vi "Emphasize Colo2r.vi"(2 "error in (no error)":errorcluster, 3 "Color":i8, 4 "Image Dst":T1, 5 "Image Src":T1) -> (0 "error out":errorcluster, 1 "Image Out":T1)   [LabVIEW 2009, in "ImageProcessing.lvlib"]
doc: "Output is a grayscaled image calculated as\n (255*X)/(R+G+B) \nwhere X is R, G or B depending on what number is showsen in color (0 = R, 1 = G, 2 = B)."
uses:
  ImageProcessing.lvlib
  <vilib>/vision/Image Controls.llb/IMAQ Image.ctl
  <vilib>/Analysis/Matrix/Numeric/Conversions/Matrix To Array - RM.vi
  <vilib>/Analysis/Matrix/Numeric/Multiply/Multiply - RM,R.vi
  <vilib>/Analysis/Matrix/Numeric/Add/Add - RM,RM.vi
  <vilib>/Analysis/Matrix/Numeric/Conversions/Array To Matrix - RA2.vi
  <vilib>/Analysis/Matrix/NI_Matrix.lvlib
  <vilib>/vision/NI_Vision_Development_Module.lvlib
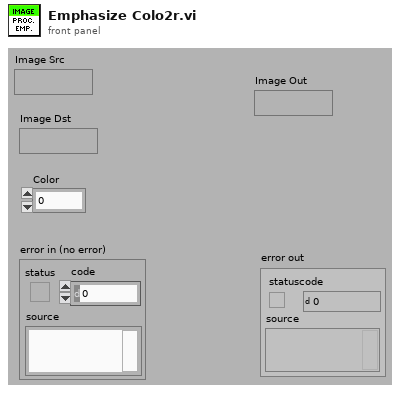
[diagram p1: front panel]
types:
  T1 = typedef "IMAQ Image.ctl" = refnum<image>
  T2 = typedef "NI_Matrix.lvlib/RealMatrix.ctl" = dbl[][]
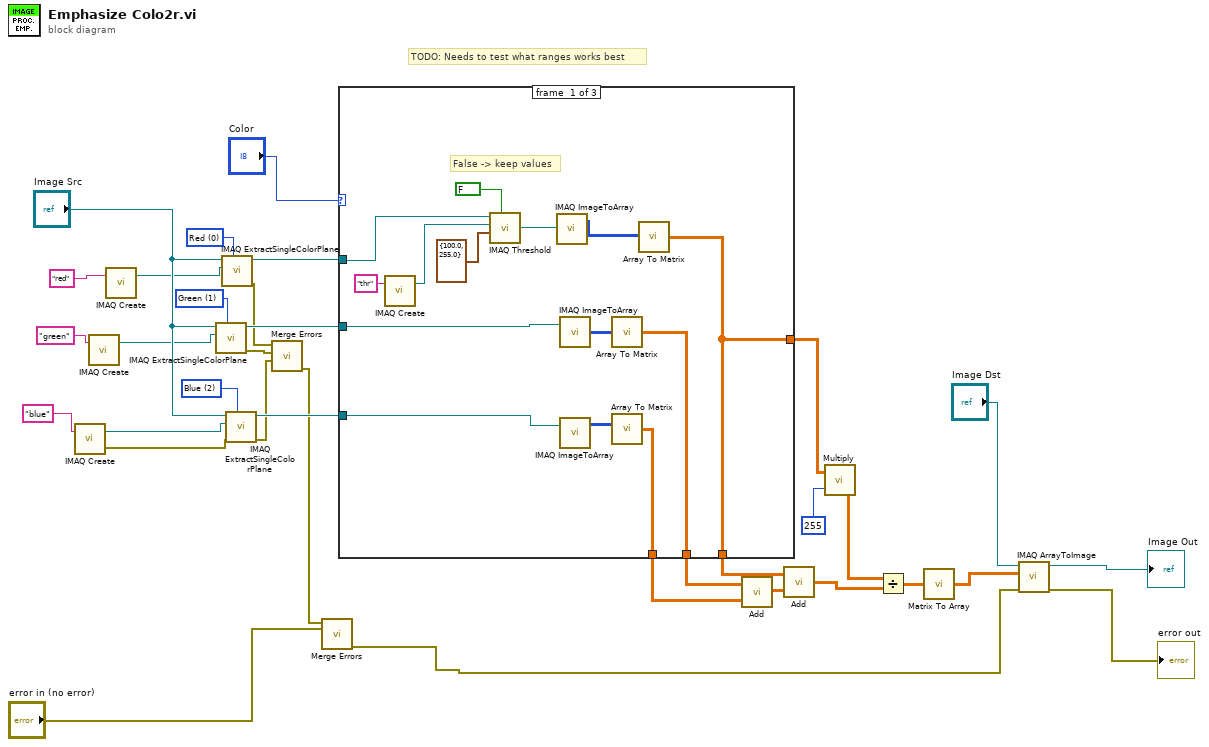
[diagram p0: block diagram]
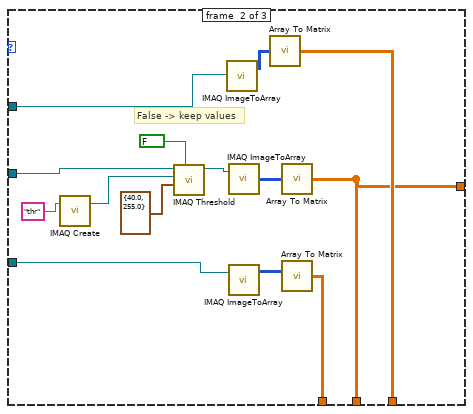
[diagram p2: hidden frame]
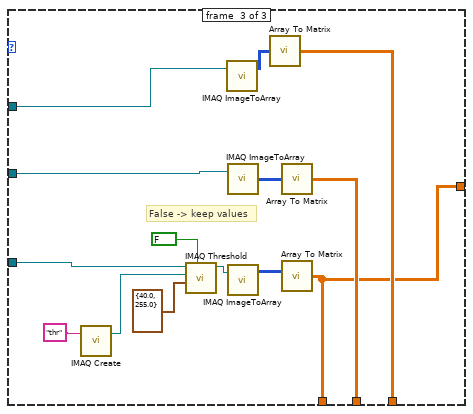
[diagram p3: hidden frame]
diagram:
  w22 = 2 items=["Red", "Green", "Blue", "Hue", "Saturation", "Luminance", "Value", "Intensity"] ("Color Plane")
  w21 = 1 items=["Red", "Green", "Blue", "Hue", "Saturation", "Luminance", "Value", "Intensity"] ("Color Plane")
  w20 = 0 items=["Red", "Green", "Blue", "Hue", "Saturation", "Luminance", "Value", "Intensity"] ("Color Plane")
  # "TODO: Needs to test what ranges works best"
  n1 = call "IMAQ Create"("Image Name"="blue") -> ("New Image"=w16:T1, "error out"=w10:errorcluster)  [unwired: 3 in, 1 out]
  n2 = call "IMAQ Create"("Image Name"="green") -> ("New Image"=w17:T1)  [unwired: 3 in, 2 out]
  n3 = call "IMAQ Create"("Image Name"="red") -> ("New Image"=w18:T1)  [unwired: 3 in, 2 out]
  n4 = call "IMAQ ExtractSingleColorPlane"("Color Plane"=w21, "Image Dst"=w17, "Image Src"="Image Src") -> ("error out"=w8:errorcluster, "Image Dst Out"=w15:T1)  [unwired: 7 in]
  n5 = call "IMAQ ExtractSingleColorPlane"("Color Plane"=w20, "Image Dst"=w18, "Image Src"="Image Src") -> ("error out"=w7:errorcluster, "Image Dst Out"=w3:T1)  [unwired: 7 in]
  n6 = call "IMAQ ExtractSingleColorPlane"("Color Plane"=w22, "error in (no error)"=w10, "Image Dst"=w16, "Image Src"="Image Src") -> ("error out"=w9:errorcluster, "Image Dst Out"=w14:T1)  [unwired: 6 in]
  n7 = call <vilib>:"Merge Errors.vi"("error in 3 (no error)"=w9, "error in 2 (no error)"=w8, "error in 1 (no error)"=w7) -> ("error out"=w4:errorcluster)  [unwired: 4 in]
  n8 = call <vilib>:"Merge Errors.vi"("error in 2 (no error)"="error in (no error)", "error in 1 (no error)"=w4) -> ("error out"=w5:errorcluster)  [unwired: 5 in]
  n9 = case shown="..0" "Color" {
    tunnel: [w38 w56 w70] -> w24
    tunnel: w3 -> [w39 w55 w63]
    tunnel: w15 -> [w45 w49 w75]
    tunnel: w14 -> [w42 w59 w64]
    tunnel: [w48 w62 w70] -> w11
    tunnel: [w47 w56 w76] -> w12
    tunnel: [w38 w58 w72] -> w13
    frame #0 {
      # "False -> keep values"
      n10 = call "IMAQ Create"("Image Name"="thr") -> ("New Image"=w40:T1)  [unwired: 3 in, 2 out]
      n11 = call "IMAQ Threshold"("Keep/Replace Value (Replace)"=FALSE, "Range"=cluster{"Lower value":sgl, "Upper value":sgl} {"Lower value"=100.0, "Upper value"=255.0}, "Image Dst"=w40, "Image Src"=w39) -> ("Image Dst Out"=w36:T1)  [unwired: 6 in, 1 out]
      n12 = call "IMAQ ImageToArray"("Image"=w36) -> ("Image Pixels (U8)"=w35:u8[][])  [unwired: 3 in, 4 out]
      n13 = call "IMAQ ImageToArray"("Image"=w45) -> ("Image Pixels (U8)"=w44:u8[][])  [unwired: 3 in, 4 out]
      n14 = call "IMAQ ImageToArray"("Image"=w42) -> ("Image Pixels (U8)"=w43:u8[][])  [unwired: 3 in, 4 out]
      n15 = call-poly <vilib>:"Array To Matrix.vi"("Real 2D Array"=w44) -> ("Real Matrix"=w47:T2)
      n16 = call-poly <vilib>:"Array To Matrix.vi"("Real 2D Array"=w43) -> ("Real Matrix"=w48:T2)
      n17 = call-poly <vilib>:"Array To Matrix.vi"("Real 2D Array"=w35) -> ("Real Matrix"=w38:T2)
    }
    frame #1 {
      # "False -> keep values"
      n18 = call "IMAQ Create"("Image Name"="thr") -> ("New Image"=w52:T1)  [unwired: 3 in, 2 out]
      n19 = call "IMAQ Threshold"("Keep/Replace Value (Replace)"=FALSE, "Range"=cluster{"Lower value":sgl, "Upper value":sgl} {"Lower value"=40.0, "Upper value"=255.0}, "Image Dst"=w52, "Image Src"=w49) -> ("Image Dst Out"=w50:T1)  [unwired: 6 in, 1 out]
      n20 = call "IMAQ ImageToArray"("Image"=w55) -> ("Image Pixels (U8)"=w57:u8[][])  [unwired: 3 in, 4 out]
      n21 = call "IMAQ ImageToArray"("Image"=w50) -> ("Image Pixels (U8)"=w61:u8[][])  [unwired: 3 in, 4 out]
      n22 = call "IMAQ ImageToArray"("Image"=w59) -> ("Image Pixels (U8)"=w60:u8[][])  [unwired: 3 in, 4 out]
      n23 = call-poly <vilib>:"Array To Matrix.vi"("Real 2D Array"=w57) -> ("Real Matrix"=w58:T2)
      n24 = call-poly <vilib>:"Array To Matrix.vi"("Real 2D Array"=w61) -> ("Real Matrix"=w56:T2)
      n25 = call-poly <vilib>:"Array To Matrix.vi"("Real 2D Array"=w60) -> ("Real Matrix"=w62:T2)
    }
    frame #2 {
      # "False -> keep values"
      n26 = call "IMAQ Create"("Image Name"="thr") -> ("New Image"=w67:T1)  [unwired: 3 in, 2 out]
      n27 = call "IMAQ Threshold"("Keep/Replace Value (Replace)"=FALSE, "Range"=cluster{"Lower value":sgl, "Upper value":sgl} {"Lower value"=40.0, "Upper value"=255.0}, "Image Dst"=w67, "Image Src"=w64) -> ("Image Dst Out"=w65:T1)  [unwired: 6 in, 1 out]
      n28 = call "IMAQ ImageToArray"("Image"=w63) -> ("Image Pixels (U8)"=w71:u8[][])  [unwired: 3 in, 4 out]
      n29 = call "IMAQ ImageToArray"("Image"=w75) -> ("Image Pixels (U8)"=w74:u8[][])  [unwired: 3 in, 4 out]
      n30 = call "IMAQ ImageToArray"("Image"=w65) -> ("Image Pixels (U8)"=w73:u8[][])  [unwired: 3 in, 4 out]
      n31 = call-poly <vilib>:"Array To Matrix.vi"("Real 2D Array"=w71) -> ("Real Matrix"=w72:T2)
      n32 = call-poly <vilib>:"Array To Matrix.vi"("Real 2D Array"=w74) -> ("Real Matrix"=w76:T2)
      n33 = call-poly <vilib>:"Array To Matrix.vi"("Real 2D Array"=w73) -> ("Real Matrix"=w70:T2)
    }
  }
  n34 = call-poly <vilib>:"Add.vi"("Real Matrix B"=w11, "Real Matrix A"=w12) -> ("A + B"=w31:T2)
  n35 = call-poly <vilib>:"Add.vi"("Real Matrix B"=w31, "Real Matrix A"=w13) -> ("A + B"=w29:T2)
  n36 = call-poly <vilib>:"Multiply.vi"("Real Scalar c"=255, "Real Matrix A"=w24) -> ("A * c"=w28:T2)
  n37 = Divide(x=w28, y=w29) -> (x/y=w1:T2)
  n38 = call-poly <vilib>:"Matrix To Array.vi"("Real Matrix"=w1) -> ("Real 2D Array"=w27:dbl[][])
  n39 = call "IMAQ ArrayToImage"("error in (no error)"=w5, "Image Pixels (U8)"=w27, "Image"="Image Dst") -> ("error out"=→"error out":errorcluster, "Image Out"=→"Image Out":T1)  [unwired: 7 in]
